vi "1Dto1DSearchА.vi"(8 "Array 2":u64[](array[numeric]), 11 "Array 1":u64[](array[numeric])) -> (0 "UnMatch el cnt":u64, 1 "Match El cnt":u64, 2 "UnMatch Elements":u64[](array[numeric]), 3 "Match Elements":u64[](array[numeric]))   [LabVIEW 2023]
panel:
  # "Търси съвпадения на елементите от Array 2 в Array 1. Извежда съвпадащите и не съвпадащите елементи в отделни масиви"
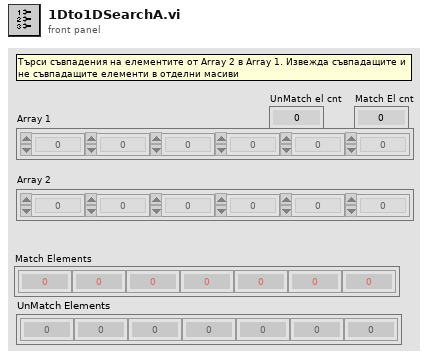
[diagram p1: front panel]
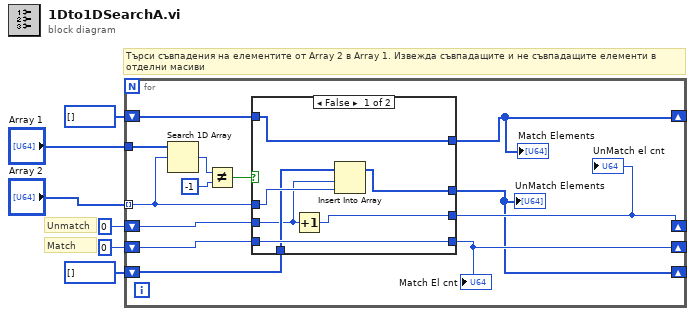
[diagram p0: block diagram]
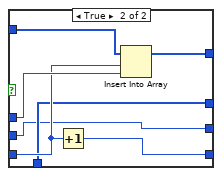
[diagram p2: hidden frame]
diagram:
  # "Търси съвпадения на елементите от Array 2 в Array 1. Извежда съвпадащите и не съвпадащите елементи в отделни масиви"
  # "Match"
  # "Unmatch"
  n1 = for {
    tunnel: "Array 1" -> [w19]
    tunnel: "Array 2" -> [w13] mode=indexing
    shift-right: [w15] -> _
    shift-left: u64 0 -> [w14]
    shift-right: [w12] -> _
    shift-left: u64[] [] -> [w11]
    shift-right: [w10] -> _
    shift-left: u64 0 -> [w9]
    shift-right: [w8] -> _
    shift-left: u64[] [] -> [w7]
    n2 = Search 1D Array(1D array=w19, element=w13) -> (index of element=w18:i32)  [unwired: 1 in]
    n3 = Not Equal?(x=w18, y=-1) -> (x != y?=w16:bool)
    n4 = case shown="False" w16 {
      tunnel: [w26 w33] -> w15
      tunnel: w14 -> [w26 w29]
      tunnel: w13 -> [w24 w32]
      tunnel: [w25 w31] -> w12
      tunnel: w11 -> [w25 w30]
      tunnel: [w23 w27] -> w10
      tunnel: w9 -> [w20 w27]
      tunnel: [w22 w28] -> w8
      tunnel: w7 -> [w21 w28]
      frame False {
        n5 = Increment(x=w20) -> (x+1=w23:u64)
        n6 = Insert Into Array "Insert Into Array"(array=w21, index=w20, new element=w24) -> (w22:u64[])
      }
      frame True {
        n7 = Increment(x=w29) -> (x+1=w33:u64)
        n8 = Insert Into Array "Insert Into Array"(array=w30, index=w29, new element=w32) -> (w31:u64[])
      }
    }
    "Match El cnt" <- w15
    "Match Elements" <- w12
    "UnMatch el cnt" <- w10
    "UnMatch Elements" <- w8
  }
